vi "Retreive Initial Load Cell.vi"(8 "error in (no error)":errorcluster, 11 "Model in":refnum<class "Model.lvclass">) -> (0 "error out":errorcluster, 1 "Encoder Value":i32, 2 "Load Cell Reading":dbl, 3 "Model out":refnum<class "Model.lvclass">)   [LabVIEW 2016, in "Model.lvclass"]
uses:
  Model.lvclass
  Model.lvclass/Model.ctl
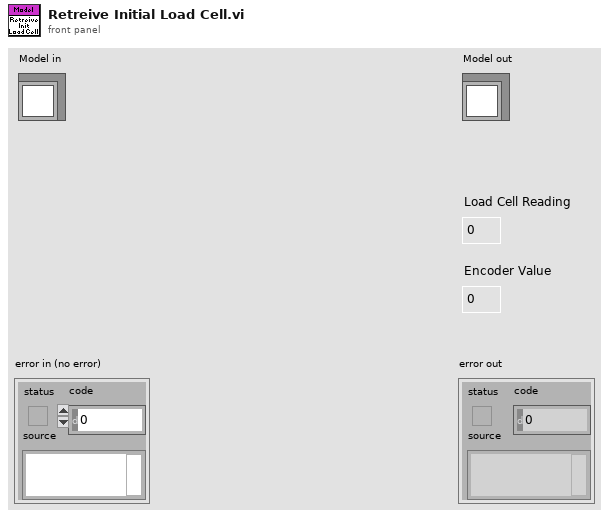
[diagram p1: front panel]
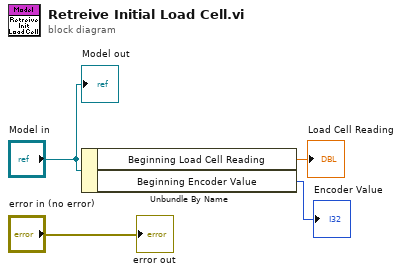
[diagram p0: block diagram]
diagram:
  n1 = Unbundle By Name("Model in") -> ("Beginning Load Cell Reading"=→"Load Cell Reading":dbl, "Beginning Encoder Value"=→"Encoder Value":i32)
  "error out" <- "error in (no error)"
  "Model out" <- "Model in"
